vi "Intake Get.vi"(1 "Gripper":dbl, 2 "Arm State":bool) -> ()   [LabVIEW 2013]
uses:
  Intake Global.vi
panel:
  # "0 < Gripper - Intake\n0 = Gripper - stop\n0 > Gripper - Eject"
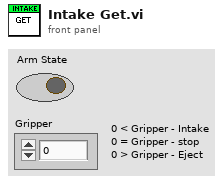
[diagram p1: front panel]
types:
  T1 = typedef "WPI_RelayValue.ctl" = enum16{"Off", "On", "Forward", "Reverse"}
  T2 = typedef "WPI_SolenoidValue.ctl" = enum16{"Off", "On", "Forward", "Reverse"}
  T3 = cluster{"Arm State":bool, "Gripper In":bool, "Gripper Out":bool, "Gripper Execution":T1, "Arm Execution":T2, "Middle MS":bool, "Middle Stop":bool}
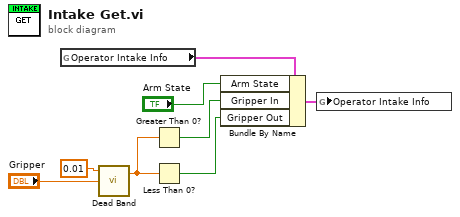
[diagram p0: block diagram]
diagram:
  n1 = global read "Intake Global.vi" "Operator Intake Info"() -> (w8:T3)
  n2 = call "Dead Band.vi"("Axis 1 In"="Gripper", "Dead Band"=0.01) -> ("Axis 1 Out"=w2:dbl)  [unwired: 1 in, 1 out]
  n3 = Greater Than 0?(x=w2) -> (x > 0?=w3:bool)
  n4 = Less Than 0?(x=w2) -> (x < 0?=w1:bool)
  n5 = Bundle By Name(cluster=w8, "Arm State"="Arm State", "Gripper In"=w3, "Gripper Out"=w1) -> (w7:T3)
  n6 = global write "Intake Global.vi" "Operator Intake Info"(w7) -> ()
